vi "n_fact_SUB.vi"(1 "n":dbl) -> (0 "n!":dbl)   [LabVIEW 2026]
panel:
  in  "const":dbl
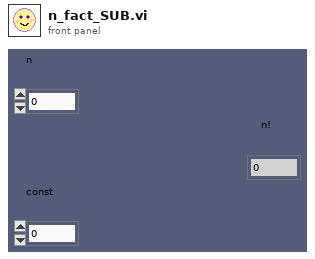
[diagram p1: front panel]
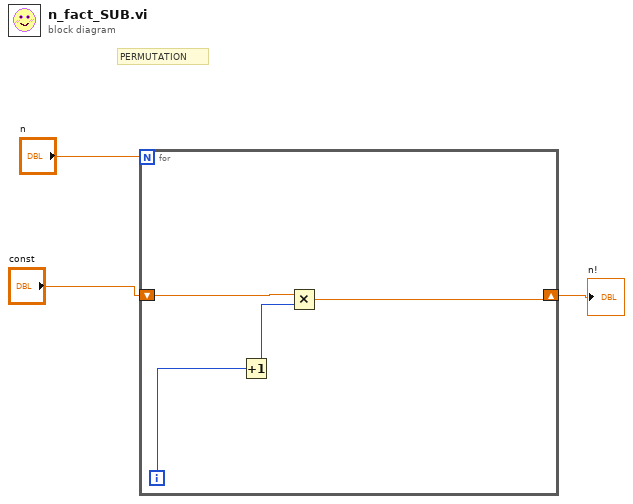
[diagram p0: block diagram]
diagram:
  # "PERMUTATION"
  n1 = for {
    N: "n" -> [_]
    shift-right: [w4] -> w1
    shift-left: "const" -> [w7]
    i -> [w6]
    n2 = Increment(x=w6) -> (x+1=w5:i32)
    n3 = Multiply(x=w7, y=w5) -> (x*y=w4:dbl)
  }
  "n!" <- w1
